vi "ERIO RT Update Supervisory Variables.vi"(6 "Server Update":bool, 8 "error in (no error)":errorcluster, 9 "AWS Variables In":T1, 10 "Secret Key":string, 11 "EEISysLink.lvclass In":refnum<class "EEISysLink.lvclass">) -> (0 "error out":errorcluster, 1 "AWS Variables Out":T1, 3 "EEISysLink.lvclass Out":refnum<class "EEISysLink.lvclass">, 4 "Supervisory Variables":T2={"Alarm Threshold"=0.0, "Shutdown"=FALSE, "Enable SNS Alarm"=FALSE, "Enable SNS Stage Notification"=FALSE, "Enable SQS Notification"=FALSE, "Enable S3 TDMS Signal Capture"=FALSE, "Enable SystemLink Signal Capture"=FALSE, "Capture Signal"=FALSE, "Server Update"=FALSE, "AWS Access Key"="AKIAINLDO2Y2PDFEWDOQ", "AWS Secret Key"="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", "Phone Number"="+15037066913", "Region"=enum."us-west-2", "AWS SQS Queue"="mynicloud-demotest2", "AWS S3 Bucket"="mynicloud-demotest2"})   [LabVIEW 2017]
doc: "Update all the supervisory variables in preparation of the next control iteration. \n\nJames Tillett P.E.\nEndeavor Engineering Inc.\nwww.endeavoreng.com"
uses:
  Class EEISysLink/EEISysLink.lvclass
  Controls/ERIO Supervisory Variables.ctl
  <vilib>/AWS Toolkit/Core/HTTP Request/Region.ctl
  Controls/ERIO AWS Toolkit Variables.ctl
  <vilib>/AWS Toolkit/SQS/Queue/Queue.lvclass
  <vilib>/AWS Toolkit/SNS/Phone Number/Phone Number.lvclass
  <vilib>/AWS Toolkit/S3/Bucket/Bucket.lvclass
  Class EEISysLink/Controls/SL Tag Scope.ctl
  Class EEISysLink/Controls/SL Tag Type.ctl
  <vilib>/AWS Toolkit/Core/HTTP Request/HTTP Request.lvclass
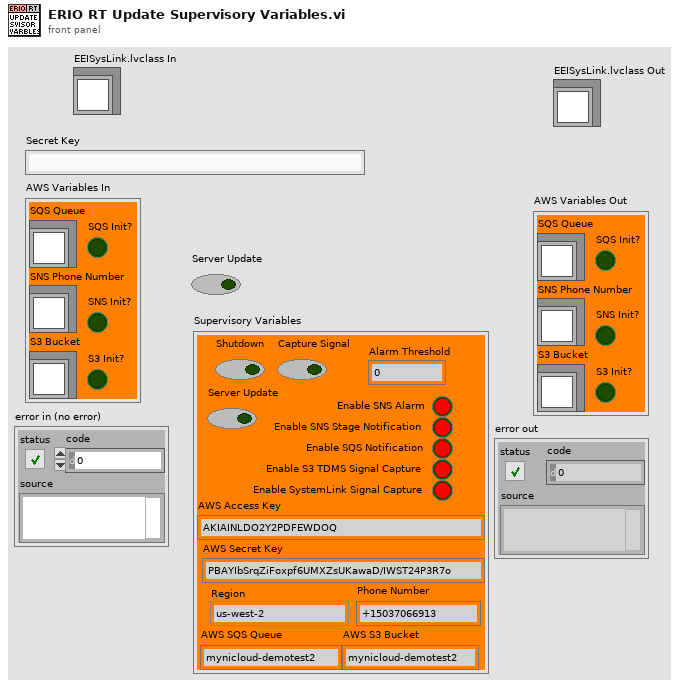
[diagram p1: front panel]
types:
  T1 = typedef "ERIO AWS Toolkit Variables.ctl" = cluster{"SQS Queue":refnum<class "Queue.lvclass">, "SNS Phone Number":refnum<class "Phone Number.lvclass">, "S3 Bucket":refnum<class "Bucket.lvclass">, "SQS Init?":bool, "S3 Init?":bool, "SNS Init?":bool}
  T2 = typedef "ERIO Supervisory Variables.ctl" = cluster{"Alarm Threshold":dbl, "Shutdown":bool, "Enable SNS Alarm":bool, "Enable SNS Stage Notification":bool, "Enable SQS Notification":bool, "Enable S3 TDMS Signal Capture":bool, "Enable SystemLink Signal Capture":bool, "Capture Signal":bool, "Server Update":bool, "AWS Access Key":string, "AWS Secret Key":string, "Phone Number":string, "Region":T3, "AWS SQS Queue":string, "AWS S3 Bucket":string}
  T3 = typedef "NI_AWS_Core.lvlib/HTTP Request.lvclass/Region.ctl" = enum16{"us-east-1", "us-east-2", "us-west-1", "us-west-2", "ap-northeast-1", "ap-northeast-2", "ap-southeast-1", "ap-southeast-2", "ca-central-1", "eu-central-1", "eu-west-1", "eu-west-2", "sa-east-1"}
  T4 = typedef "EEISysLink.lvclass/SL Tag Scope.ctl" = enum16{"Local", "Server"}
  T5 = typedef "EEISysLink.lvclass/SL Tag Type.ctl" = enum16{"All", "Supervisor", "Worker"}
  T6 = typedef "SL Tag Value.ctl" = cluster{"Value":variant, "Time Stamp":timestamp, "Tag Data Type":T7, "Name":string}
  T7 = typedef "EEISysLink.lvclass/SL Tag Data Type.ctl" = enum16{"Double", "Integer", "String", "Boolean", "Waveform"}
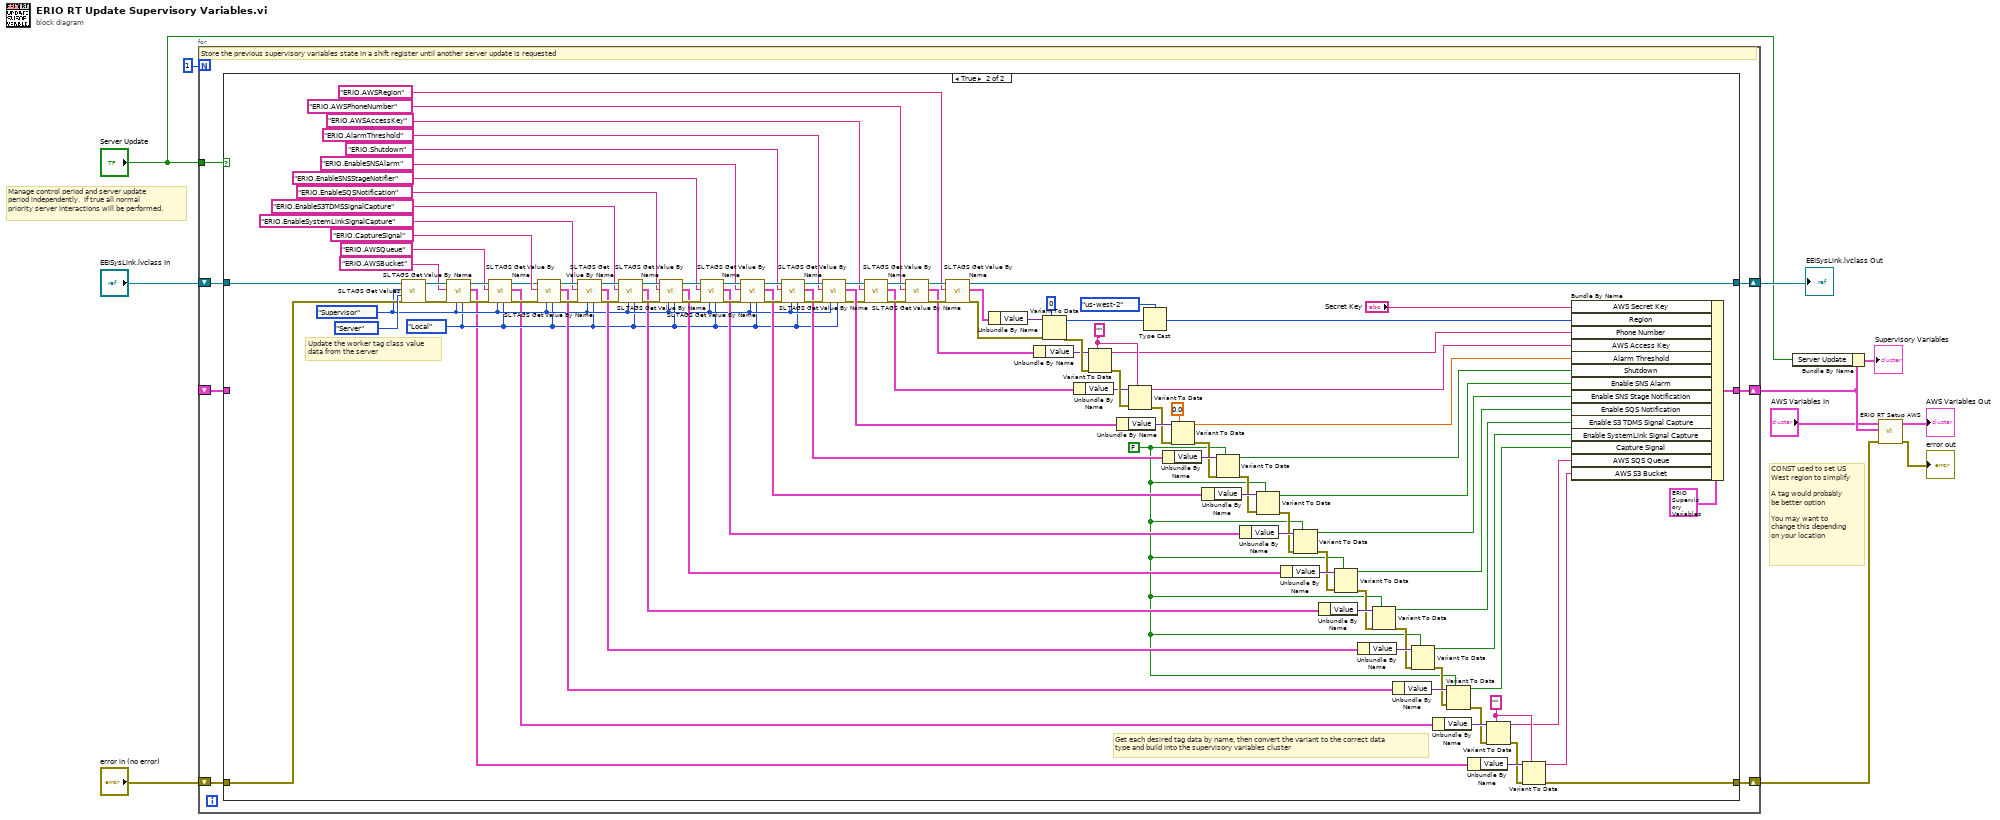
[diagram p0: block diagram]
diagram:
  # "CONST used to set US\nWest region to simplify\n\nA tag would probably\nbe better option\n\nYou may want to \nchange this depending\non your location"
  # "Manage control period and server update\nperiod independently.  If true all normal \npriority server interactions will be performed."
  n1 = for {
    N: 1 -> [_]
    shift-right: [w15] -> w1
    shift-left: "error in (no error)" -> [w17]
    shift-right: [w16] -> w5
    shift-left: _ -> [w12]
    shift-right: [w14] -> w9
    shift-left: "EEISysLink.lvclass In" -> [w18]
    tunnel: "Server Update" -> [w13]
    # "Store the previous supervisory variables state in a shift register until another server update is requested"
    n2 = case shown="True" w13 {
      tunnel: w18 -> [w19 w128]
      tunnel: w17 -> [w21 w127]
      tunnel: [w20 w23] -> w16
      tunnel: [w21 w22] -> w15
      tunnel: [w19 w54] -> w14
      tunnel: w12 -> [w20 _]
      frame False {
        # "No server update requested so just return the previous state variables stored in the shift register"
      }
      frame True {
        w30 = ""
        w47 = ""
        w78 = FALSE
        w37 = SL_Tag_Scope."Local" ("Tag Scope")
        w38 = SL_Tag_Type."Supervisor" ("Tag Type")
        # "Update the worker tag class value\ndata from the server"
        # "Get each desired tag data by name, then convert the variant to the correct data\ntype and build into the supervisory variables cluster"
        n3 = call-dynamic "SL TAGS Get Values.vi"("error in (no error)"=w127, "Tag Scope"=SL_Tag_Scope."Server", "Tag Type"=w38, "EEISysLink in"=w128) -> ("error out"=w41:errorcluster, "EEISysLink out"=w42:refnum<class "EEISysLink.lvclass">)  [unwired: 5 in, 1 out]
        n4 = call-dynamic "SL TAGS Get Value By Name.vi"("Tag Scope"=w37, "Tag Type"=w38, "error in (no error)"=w41, "Tag Name"="ERIO.AWSBucket", "EEISysLink in"=w42) -> ("error out"=w40:errorcluster, "Tag Value"=w28:T6, "EEISysLink out"=w44:refnum<class "EEISysLink.lvclass">)  [unwired: 3 in, 1 out]
        n5 = call-dynamic "SL TAGS Get Value By Name.vi"("Tag Scope"=w37, "Tag Type"=w38, "error in (no error)"=w40, "Tag Name"="ERIO.AWSQueue", "EEISysLink in"=w44) -> ("error out"=w39:errorcluster, "Tag Value"=w29:T6, "EEISysLink out"=w43:refnum<class "EEISysLink.lvclass">)  [unwired: 3 in, 1 out]
        n6 = call-dynamic "SL TAGS Get Value By Name.vi"("Tag Scope"=w37, "Tag Type"=w38, "error in (no error)"=w39, "Tag Name"="ERIO.CaptureSignal", "EEISysLink in"=w43) -> ("error out"=w118:errorcluster, "Tag Value"=w111:T6, "EEISysLink out"=w125:refnum<class "EEISysLink.lvclass">)  [unwired: 3 in, 1 out]
        n7 = call-dynamic "SL TAGS Get Value By Name.vi"("Tag Scope"=w37, "Tag Type"=w38, "error in (no error)"=w118, "Tag Name"="ERIO.EnableSystemLinkSignalCapture", "EEISysLink in"=w125) -> ("error out"=w117:errorcluster, "Tag Value"=w94:T6, "EEISysLink out"=w124:refnum<class "EEISysLink.lvclass">)  [unwired: 3 in, 1 out]
        n8 = call-dynamic "SL TAGS Get Value By Name.vi"("Tag Scope"=w37, "Tag Type"=w38, "error in (no error)"=w117, "Tag Name"="ERIO.EnableS3TDMSSignalCapture", "EEISysLink in"=w124) -> ("error out"=w116:errorcluster, "Tag Value"=w93:T6, "EEISysLink out"=w123:refnum<class "EEISysLink.lvclass">)  [unwired: 3 in, 1 out]
        n9 = call-dynamic "SL TAGS Get Value By Name.vi"("Tag Scope"=w37, "Tag Type"=w38, "error in (no error)"=w116, "Tag Name"="ERIO.EnableSQSNotification", "EEISysLink in"=w123) -> ("error out"=w115:errorcluster, "Tag Value"=w92:T6, "EEISysLink out"=w122:refnum<class "EEISysLink.lvclass">)  [unwired: 3 in, 1 out]
        n10 = call-dynamic "SL TAGS Get Value By Name.vi"("Tag Scope"=w37, "Tag Type"=w38, "error in (no error)"=w115, "Tag Name"="ERIO.EnableSNSStageNotifier", "EEISysLink in"=w122) -> ("error out"=w114:errorcluster, "Tag Value"=w91:T6, "EEISysLink out"=w121:refnum<class "EEISysLink.lvclass">)  [unwired: 3 in, 1 out]
        n11 = call-dynamic "SL TAGS Get Value By Name.vi"("Tag Scope"=w37, "Tag Type"=w38, "error in (no error)"=w114, "Tag Name"="ERIO.EnableSNSAlarm", "EEISysLink in"=w121) -> ("error out"=w113:errorcluster, "Tag Value"=w90:T6, "EEISysLink out"=w120:refnum<class "EEISysLink.lvclass">)  [unwired: 3 in, 1 out]
        n12 = call-dynamic "SL TAGS Get Value By Name.vi"("Tag Scope"=w37, "Tag Type"=w38, "error in (no error)"=w113, "Tag Name"="ERIO.Shutdown", "EEISysLink in"=w120) -> ("error out"=w112:errorcluster, "Tag Value"=w89:T6, "EEISysLink out"=w119:refnum<class "EEISysLink.lvclass">)  [unwired: 3 in, 1 out]
        n13 = call-dynamic "SL TAGS Get Value By Name.vi"("Tag Scope"=w37, "Tag Type"=w38, "error in (no error)"=w112, "Tag Name"="ERIO.AlarmThreshold", "EEISysLink in"=w119) -> ("error out"=w59:errorcluster, "Tag Value"=w88:T6, "EEISysLink out"=w60:refnum<class "EEISysLink.lvclass">)  [unwired: 3 in, 1 out]
        n14 = call-dynamic "SL TAGS Get Value By Name.vi"("error in (no error)"=w59, "Tag Name"="ERIO.AWSAccessKey", "EEISysLink in"=w60) -> ("error out"=w63:errorcluster, "Tag Value"=w57:T6, "EEISysLink out"=w61:refnum<class "EEISysLink.lvclass">)  [unwired: 5 in, 1 out]
        n15 = call-dynamic "SL TAGS Get Value By Name.vi"("error in (no error)"=w63, "Tag Name"="ERIO.AWSPhoneNumber", "EEISysLink in"=w61) -> ("error out"=w64:errorcluster, "Tag Value"=w56:T6, "EEISysLink out"=w62:refnum<class "EEISysLink.lvclass">)  [unwired: 5 in, 1 out]
        n16 = call-dynamic "SL TAGS Get Value By Name.vi"("error in (no error)"=w64, "Tag Name"="ERIO.AWSRegion", "EEISysLink in"=w62) -> ("error out"=w58:errorcluster, "Tag Value"=w55:T6, "EEISysLink out"=w54:refnum<class "EEISysLink.lvclass">)  [unwired: 5 in, 1 out]
        n17 = Unbundle By Name(w55) -> ("Value"=w67:variant)
        n18 = Unbundle By Name(w56) -> ("Value"=w66:variant)
        n19 = Variant To Data(error in=w58, type=u16 0, Variant=w67) -> (data=w48:u16, error out=w68:errorcluster)
        n20 = Unbundle By Name(w57) -> ("Value"=w65:variant)
        n21 = Variant To Data(error in=w68, type=w47, Variant=w66) -> (data=w45:string, error out=w69:errorcluster)
        n22 = Unbundle By Name(w88) -> ("Value"=w95:variant)
        n23 = Variant To Data(error in=w69, type=w47, Variant=w65) -> (data=w24:string, error out=w53:errorcluster)
        n24 = Type Cast(type=Region."us-west-2" ("AWS Region"), x=w48) -> (*(type *) &x=w46:T3)
        n25 = Unbundle By Name(w89) -> ("Value"=w96:variant)
        n26 = Variant To Data(error in=w53, type=0.0, Variant=w95) -> (data=w79:dbl, error out=w87:errorcluster)
        n27 = Unbundle By Name(w90) -> ("Value"=w97:variant)
        n28 = Variant To Data(error in=w87, type=w78, Variant=w96) -> (data=w77:bool, error out=w86:errorcluster)
        n29 = Unbundle By Name(w91) -> ("Value"=w98:variant)
        n30 = Variant To Data(error in=w86, type=w78, Variant=w97) -> (data=w76:bool, error out=w85:errorcluster)
        n31 = Unbundle By Name(w92) -> ("Value"=w99:variant)
        n32 = Variant To Data(error in=w85, type=w78, Variant=w98) -> (data=w75:bool, error out=w84:errorcluster)
        n33 = Unbundle By Name(w93) -> ("Value"=w100:variant)
        n34 = Variant To Data(error in=w84, type=w78, Variant=w99) -> (data=w74:bool, error out=w83:errorcluster)
        n35 = Unbundle By Name(w94) -> ("Value"=w101:variant)
        n36 = Variant To Data(error in=w83, type=w78, Variant=w100) -> (data=w73:bool, error out=w82:errorcluster)
        n37 = Unbundle By Name(w111) -> ("Value"=w102:variant)
        n38 = Variant To Data(error in=w82, type=w78, Variant=w101) -> (data=w72:bool, error out=w81:errorcluster)
        n39 = Unbundle By Name(w29) -> ("Value"=w34:variant)
        n40 = Variant To Data(error in=w81, type=w78, Variant=w102) -> (data=w71:bool, error out=w32:errorcluster)
        n41 = Unbundle By Name(w28) -> ("Value"=w33:variant)
        n42 = Variant To Data(error in=w32, type=w30, Variant=w34) -> (data=w26:string, error out=w31:errorcluster)
        n43 = Variant To Data(error in=w31, type=w30, Variant=w33) -> (data=w27:string, error out=w22:errorcluster)
        n44 = Bundle By Name(cluster=T2 {"Alarm Threshold"=0.0, "Shutdown"=FALSE, "Enable SNS Alarm"=FALSE, "Enable SNS Stage Notification"=FALSE, "Enable SQS Notification"=FALSE, "Enable S3 TDMS Signal Capture"=FALSE, "Enable SystemLink Signal Capture"=FALSE, "Capture Signal"=FALSE, "Server Update"=FALSE, "AWS Access Key"="AKIAINLDO2Y2PDFEWDOQ", "AWS Secret Key"="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", "Phone Number"="+15037066913", "Region"=enum."us-west-2", "AWS SQS Queue"="mynicloud-demotest2", "AWS S3 Bucket"="mynicloud-demotest2"} ("Supervisory Variables"), "AWS Secret Key"="Secret Key", "Region"=w46, "Phone Number"=w45, "AWS Access Key"=w24, "Alarm Threshold"=w79, "Shutdown"=w77, "Enable SNS Alarm"=w76, "Enable SNS Stage Notification"=w75, "Enable SQS Notification"=w74, "Enable S3 TDMS Signal Capture"=w73, "Enable SystemLink Signal Capture"=w72, "Capture Signal"=w71, "AWS SQS Queue"=w26, "AWS S3 Bucket"=w27) -> (w23:T2)
      }
    }
  }
  "EEISysLink.lvclass Out" <- w9
  n45 = Bundle By Name(cluster=w5, "Server Update"="Server Update") -> (→"Supervisory Variables":T2)
  n46 = call "ERIO RT Setup AWS.vi"("error in (no error)"=w1, "Supervisory Variables"=w5, "AWS Variables In"="AWS Variables In") -> ("error out"=→"error out":errorcluster, "AWS Variables Out"=→"AWS Variables Out":T1)  [unwired: 7 in]
